vi "FGV Simple Register and Unregister.vi"() -> (2 "response message":string[](array[string]), 3 "response message":string[](array[string]))   [LabVIEW 2017, in "testcase-Broadcast Registry.lvclass"]
uses:
  testcase-Broadcast Registry.lvclass
  user.lib/_NEVSTOP/Communicable State Machine(CSM)/_Support/FGV-BroadcastRegistry/Operation-BroadcastRegistry.ctl
  user.lib/_NEVSTOP/Communicable State Machine(CSM)/Communicable State Machine.lvlib
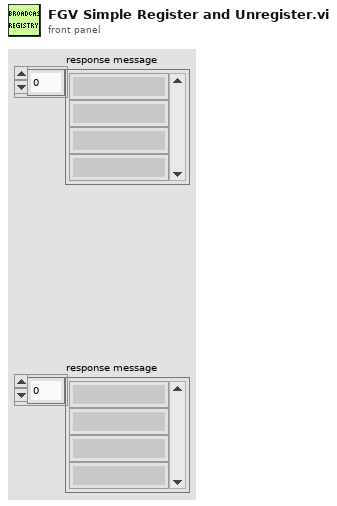
[diagram p1: front panel]
types:
  T1 = typedef "Communicable State Machine.lvlib/Operation-BroadcastRegistry.ctl" = enum16{"Delete Source Module", "Delete Target Module", "Remove Module", "Register", "Unregister", "Check", "List Status", "List Entries"}
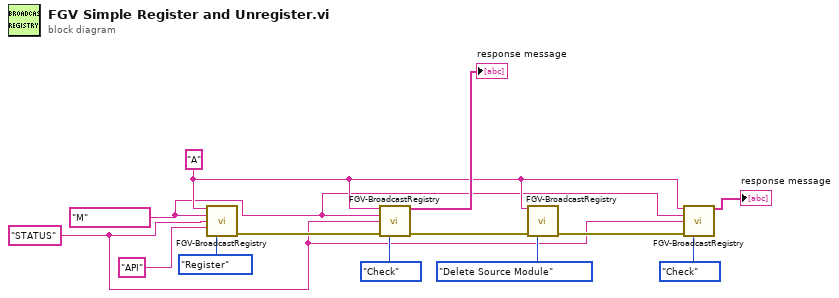
[diagram p0: block diagram]
diagram:
  w2 = "STATUS" ("Message")
  w3 = "M" ("Dest")
  w4 = "A" ("Source")
  n1 = call "FGV-BroadcastRegistry.vi"("Source"=w4, "Target"=w3, "Status"=w2, "API"="API" ("Response Message In"), "Operation"=Operation-BroadcastRegistry."Register") -> ("Error out"=w11:errorcluster)  [unwired: 9 in, 1 out]
  n2 = call "FGV-BroadcastRegistry.vi"("Source"=w4, "Target"=w3, "Status"=w2, "Error in"=w11, "Operation"=Operation-BroadcastRegistry."Check") -> ("response message"=→"response message":string[], "Error out"=w8:errorcluster)  [unwired: 9 in]
  n3 = call "FGV-BroadcastRegistry.vi"("Source"=w4, "Error in"=w8, "Operation"=Operation-BroadcastRegistry."Delete Source Module") -> ("Error out"=w5:errorcluster)  [unwired: 11 in, 1 out]
  n4 = call "FGV-BroadcastRegistry.vi"("Source"=w4, "Target"=w3, "Status"=w2, "Error in"=w5, "Operation"=Operation-BroadcastRegistry."Check") -> ("response message"=→"response message":string[])  [unwired: 9 in, 1 out]
